vi "Test PAS Write to File.vi"() -> ()   [LabVIEW 2012]
uses:
  Reusable/Switch/Switch.lvclass
  Devices/Alicat/AlicatCommBank/AlicatCommBank.lvclass
  Devices/Alicat/M/M.lvclass
  Devices/Alicat/MC/Alicat_MC.lvclass
  Devices/Alicat/Controls/Gas.ctl
  Devices/Alicat/Alicat.lvclass
  Devices/TE Cooler/TE Cooler.lvclass
  Reusable/PAS/Cell/PAS Cell.lvclass
  cPAS.lvclass
  Reusable/PAS/Main/Controls/LasLam.ctl
  Reusable/PAS/Main/Controls/Cell Condition.ctl
  <userlib>/Serialization/Deserializer/Deserializer.lvclass
  <userlib>/Serialization/Serialization Common/Serial Version.ctl
  <userlib>/Serialization/Serialization Common/Serialization Common.lvlib
  <userlib>/Serialization/JSON Deserializer/JSON Deserializer.lvclass
  <userlib>/Serialization/Serialization Common/String Contents.ctl
  <userlib>/Serialization/Formatter/Formatter.lvclass
panel:
  out "appended path":path
  out "path":path
  out "Application Directory":path
  out "class path 4":path
  out "class path 3":path
  out "class path 2":path
  out "class path":path
  out "error out":errorcluster
  out "JSON String":string
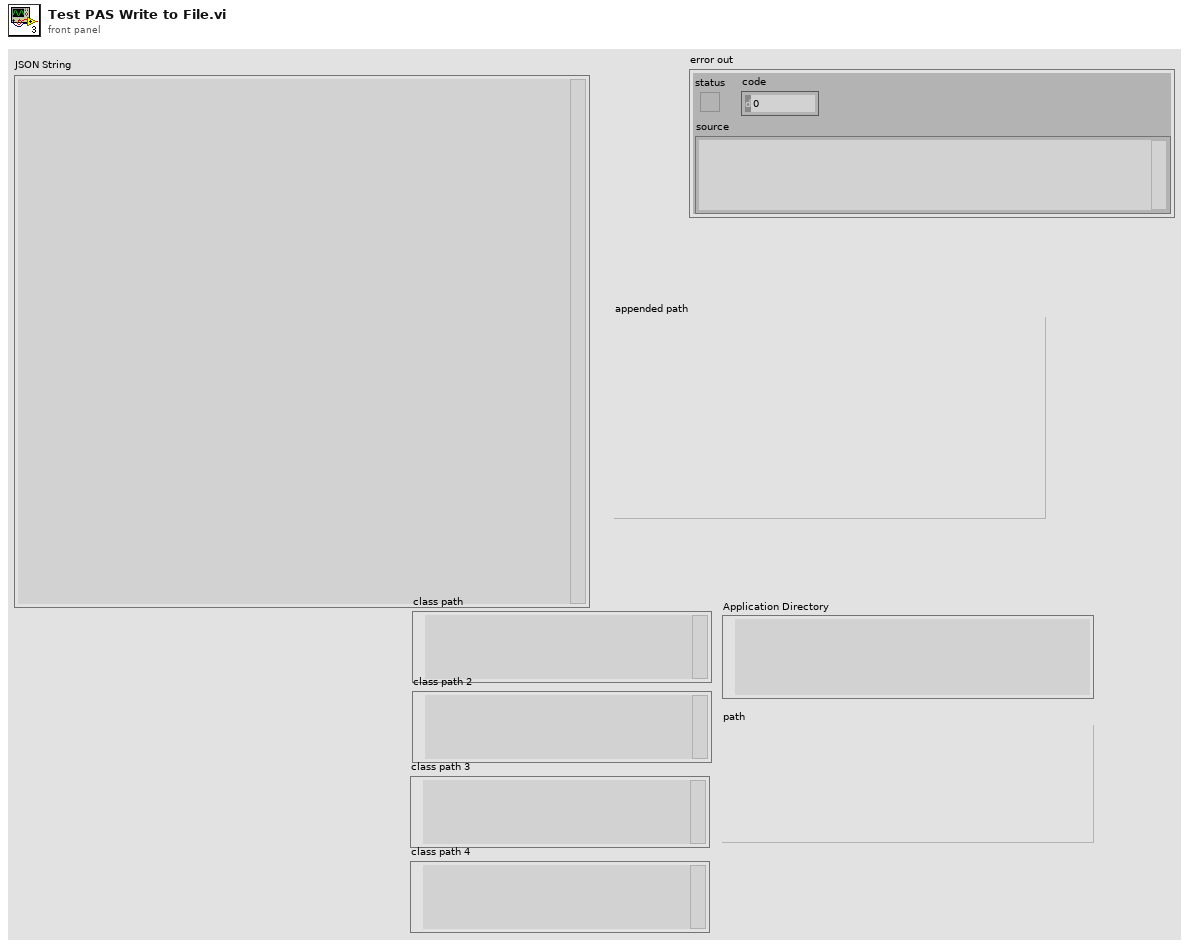
[diagram p1: front panel]
types:
  T1 = enum16{"No paths embedded", "One path with each object", "All paths with top object"}
  T2 = typedef "Serialization Common.lvlib/String Contents.ctl" = enum16{"data only", "version+data"}
  T3 = typedef "Serialization Common.lvlib/Serial Version.ctl" = cluster{"Major":u16, "Minor":u16, "Fix":u16, "Build":u16}
  T4 = typedef "Alicat.lvlib/Alicat.lvclass/Gas.ctl" = enum16{"Air", "Ar", "CH4", "CO", "CO2", "C2H6", "H2", "He", "N2", "NO", "Ne", "O2", "C3H8", "n-C4H10", "C2H2", "C2H4", "i-C2H10", "Kr", "Xe"}
  T5 = typedef "LasLam.ctl" = enum16{"405", "532", "661"}
  T6 = typedef "Cell Condition.ctl" = enum16{"Dry", "Humidified", "Denuded"}
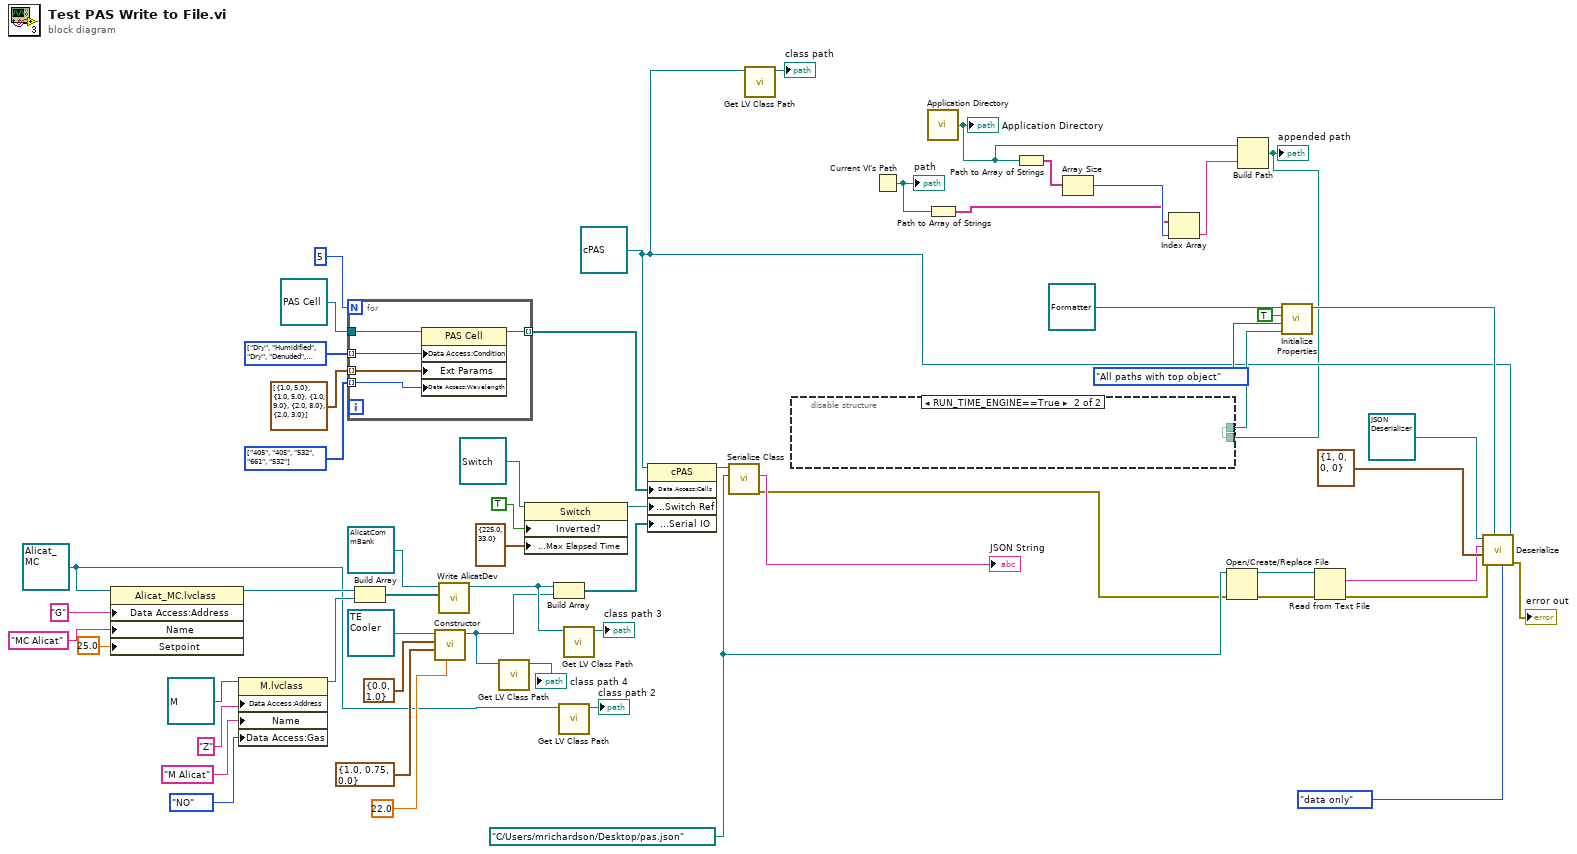
[diagram p0: block diagram]
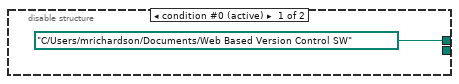
[diagram p2: hidden frame]
diagram:
  w13 = refnum<class "Alicat_MC.lvclass"> refnum ("Alicat.lvlib:Alicat_MC.lvclass")
  w54 = T5[] [enum."405", enum."405", enum."532", enum."661", enum."532"] items=["405", "532", "661"]
  w55 = T6[] [enum."Dry", enum."Humidified", enum."Dry", enum."Denuded", enum."Humidified"] items=["Dry", "Humidified", "Denuded"]
  w27 = path "C:/Users/mrichardson/Desktop/pas.json" ("file path")
  w15 = refnum<class "cPAS.lvclass"> refnum ("cPAS Server Library.lvlib:cPAS")
  n1 = property class="Alicat_MC.lvclass"(reference=w13, "Data Access:Address"="G" ("Address"), "Name"="MC Alicat", "Setpoint"=sgl 25.0) -> (reference out=w45:refnum<class "Alicat_MC.lvclass">)  [unwired: 1 in, 1 out]
  n2 = property class="M.lvclass"(reference=refnum<class "M.lvclass"> refnum ("Alicat.lvlib:M.lvclass"), "Data Access:Address"="Z" ("Address"), "Name"="M Alicat", "Data Access:Gas"=Gas."NO" ("Gas")) -> (reference out=w46:refnum<class "M.lvclass">)  [unwired: 1 in, 1 out]
  n3 = for {
    N: 5 -> [_]
    tunnel: refnum<class "PAS Cell.lvclass"> refnum ("Base PAS.lvlib:PAS Cell") -> [w63]
    tunnel: [w62] -> w57 mode=indexing
    tunnel: w55 -> [w61] mode=indexing
    tunnel: w54 -> [w60] mode=indexing
    tunnel: cluster{"slope":sgl, "zero":sgl}[] [{"slope"=1.0, "zero"=5.0}, {"slope"=1.0, "zero"=5.0}, {"slope"=1.0, "zero"=9.0}, {"slope"=2.0, "zero"=8.0}, {"slope"=2.0, "zero"=3.0}] -> [w59] mode=indexing
    n4 = property class="PAS Cell"(reference=w63, "Data Access:Condition"=w61, "Ext Params"=w59, "Data Access:Wavelength"=w60) -> (reference out=w62:refnum<class "PAS Cell.lvclass">)  [unwired: 1 in, 1 out]
  }
  n5 = Build Array(w45, w46) -> (w39:refnum<class "Alicat.lvclass">[])
  n6 = call "Constructor.vi"("TSP"=sgl 22.0, "PID Params"=cluster{"P":sgl, "I":sgl, "D":sgl} {"P"=1.0, "I"=0.75, "D"=0.0}, "Ctl Params"=cluster{"htx":sgl, "clx":sgl} {"htx"=0.0, "clx"=1.0}, "TE Cooler in"=refnum<class "TE Cooler.lvclass"> refnum ("TE Cooler.lvlib:TE Cooler.lvclass")) -> ("TE Cooler out"=w9:refnum<class "TE Cooler.lvclass">)  [unwired: 6 in, 1 out]
  n7 = call "Write AlicatDev.vi"("AlicatDev"=w39, "AlicatCommBank in"=refnum<class "AlicatCommBank.lvclass"> refnum ("Alicat.lvlib:AC Comm")) -> ("AlicatCommBank out"=w11:refnum<class "AlicatCommBank.lvclass">)  [unwired: 8 in, 1 out]
  n8 = call <vilib>:"Get LV Class Path.vi"("object"=w9) -> ("class path"=→"class path 4":path)  [unwired: 9 in, 1 out]
  n9 = property class="Switch"(reference=refnum<class "Switch.lvclass"> refnum ("Switch Ref"), "Inverted?"=TRUE, "Data Access:Max Elapsed Time"=cluster{"true":dbl, "false":dbl} {"true"=225.0, "false"=33.0} ("Max Elapsed Time")) -> (reference out=w49:refnum<class "Switch.lvclass">)  [unwired: 1 in, 1 out]
  n10 = Build Array(w11, w9) -> (w32:refnum<class "Serial IO.lvclass">[])
  n11 = call <vilib>:"Get LV Class Path.vi"("object"=w13) -> ("class path"=→"class path 2":path)  [unwired: 9 in, 1 out]
  n12 = call <vilib>:"Get LV Class Path.vi"("object"=w11) -> ("class path"=→"class path 3":path)  [unwired: 9 in, 1 out]
  n13 = property class="cPAS"(reference=w15, "Data Access:Cells"=w57, "Data Access:Switch Ref"=w49, "Data Access:Serial IO"=w32) -> (reference out=w48:refnum<class "cPAS.lvclass">)  [unwired: 1 in, 1 out]
  n14 = call-dynamic "Serialize Class.vi"("file path"=w27, "Instrument in"=w48) -> ("error out"=w24:errorcluster, "JSON String"=→"JSON String":string)  [unwired: 7 in, 1 out]
  n15 = call <vilib>:"Get LV Class Path.vi"("object"=w15) -> ("class path"=→"class path":path)  [unwired: 9 in, 1 out]
  n16 = Current VI's Path() -> (path=w7:path)
  "path" <- w7
  n17 = call <vilib>:"Application Directory.vi"() -> ("Application Directory"=w2:path)
  "Application Directory" <- w2
  n18 = Path to Array of Strings(0:w7) -> (2:w4:string[])  [unwired: 1 out]
  n19 = Path to Array of Strings(0:w2) -> (2:w6:string[])  [unwired: 1 out]
  n20 = Array Size(array=w6) -> (size(s)=w5:i32)
  n21 = Index Array(array=w4, index=w5) -> (element=w3:string)
  n22 = Open/Create/Replace File(file path (use dialog)=w27, error in=w24) -> (refnum out=w26:refnum<file>, error out=w25:errorcluster)  [unwired: 4 in, 1 out]
  n23 = Build Path(base path=w2, name or relative path=w3) -> (appended path=w1:path)
  "appended path" <- w1
  n24 = disable-structure shown="RUN_TIME_ENGINE==True" {
    disable-tunnel: [path "C:/Users/mrichardson/Documents/Web Based Version Control SW" ("Absolute Path For Dynamic Loading") w65] -> w16
    disable-tunnel: w1 -> [_ w65]
    frame condition #0 (active) {
    }
    frame condition #1 {
    }
  }
  n25 = call <userlib>:"Initialize Properties.vi"("Absolute Path For Dynamic Loading"=w16, "Path Embedding"=T1."All paths with top object", "Include all fields?"=TRUE, "Formatter in (Default Formatter)"=refnum<class "Formatter.lvclass"> refnum) -> ("Formatter out"=w19:refnum<class "Formatter.lvclass">)  [unwired: 7 in]
  n26 = Read from Text File(file (use dialog)=w26, error in=w25) -> (text=w28:string, error out=w23:errorcluster)  [unwired: 2 in, 2 out]
  n27 = call <userlib>:"Deserialize.vi"("Target Type (Serializable.lvclass)"=w15, "String Contents (data only)"=String_Contents."data only", "Formatter (defaults)"=w19, "error in (no error)"=w23, "Serial Version (1.0.0.0)"=T3 {"Major"=1, "Minor"=0, "Fix"=0, "Build"=0}, "String"=w28, "Deserializer"=refnum<class "JSON Deserializer.lvclass"> refnum ("JSON Deserializer.lvclass")) -> ("error out"=→"error out":errorcluster)  [unwired: 2 in, 2 out]
